vi "13_DC Motor_cts2cm.vi"() -> ()   [LabVIEW 2018]
uses:
  <userlib>/KNR OS 4.0 LabVIEW Toolkit/Type Definition/Resource.ctl
  <userlib>/KNR OS 4.0 LabVIEW Toolkit/Type Definition/DC Motor Port.ctl
panel:
  in  "Speed (+-100%)":dbl(slide) scale=-100.0..100.0
  in  "IP":string(combo)="172.22.11.2"
  in  "Port":T1=4 items=["DS1"=4, "DS2"=5, "DS3"=6, "DS4"=7]
  in  "Resource":T2=enum."KNRm_DDDD"
  in  "stop":bool
  in  "Enable Motor":bool
  out "Position cm":dbl
  out "Velocity (cts/sec)":dbl
  in  "Reverse?":bool
  in  "Reset":bool
  # "KNR/KNRm\nPort5=DS1\nPort6=DS2\nPort7=DS3\nPort8=DS4"
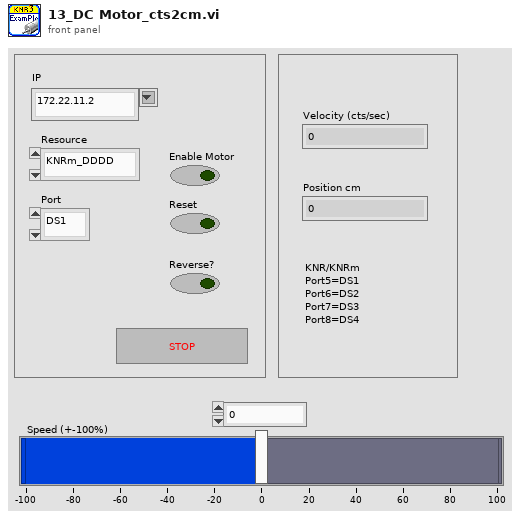
[diagram p1: front panel]
types:
  T1 = typedef "DC Motor Port.ctl" = u16
  T2 = typedef "Resource.ctl" = enum16{"KNRm_DDRC", "KNRm_DDDD", "KNRm_DDDR", "KNRm_DDDC", "KNR", "KNRm_neww"}
  T3 = typedef "KNR3 Reference.ctl" = cluster{"FPGA Session":refnum<class "FPGA Interface Base.lvclass">, "Resource":T2}
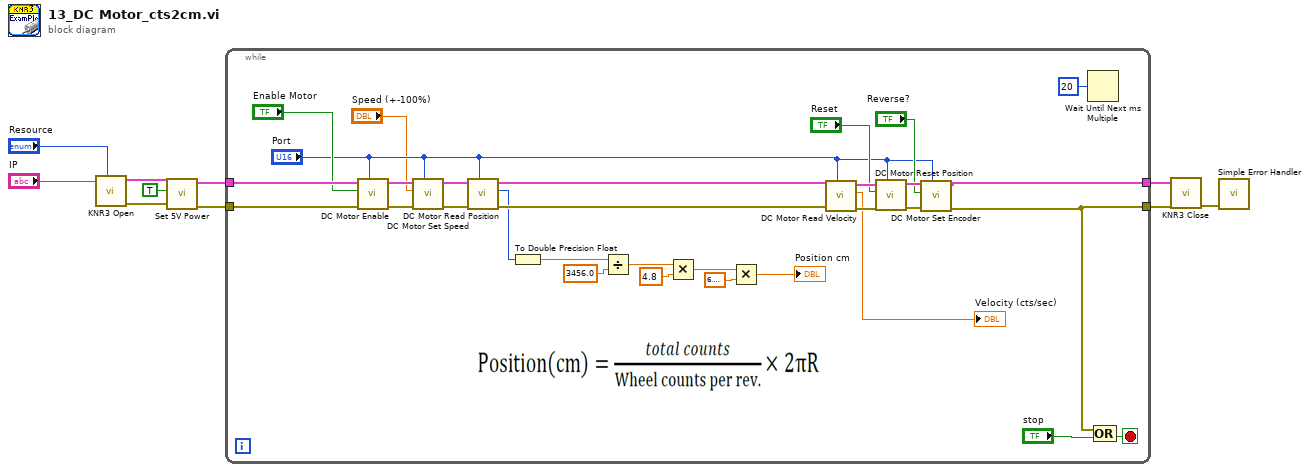
[diagram p0: block diagram]
diagram:
  n1 = call <userlib>:"KNR3 Open.vi"("Resource"="Resource", "IP"="IP") -> ("error out"=w2:errorcluster, "KNR out"=w4:T3)  [unwired: 8 in]
  n2 = call <userlib>:"Set 5V Power.vi"("error in (no error)"=w2, "5V Power(T)"=TRUE ("5V Power"), "KNR in"=w4) -> ("error out"=w8:errorcluster, "KNR out"=w9:T3)  [unwired: 7 in]
  n3 = while {
    tunnel: w9 -> [w41]
    tunnel: w8 -> [w37]
    tunnel: [w26] -> w6
    tunnel: [w27] -> w7
    stop <- w33 stop-if-true
    n4 = call <userlib>:"DC Motor Enable.vi"("Port (DS1)"="Port", "error in (no error)"=w37, "Enable Motor(F)"="Enable Motor", "KNR in"=w41) -> ("error out"=w36:errorcluster, "KNR out"=w40:T3)  [unwired: 6 in]
    n5 = call <userlib>:"DC Motor Set Speed.vi"("Port (DS1)"="Port", "error in (no error)"=w36, "Speed (+-100%)"="Speed (+-100%)", "KNR in"=w40) -> ("error out"=w35:errorcluster, "KNR out"=w39:T3)  [unwired: 6 in]
    n6 = call <userlib>:"DC Motor Read Position.vi"("Port (DS1)"="Port", "error in (no error)"=w35, "KNR in"=w39) -> ("error out"=w30:errorcluster, "Position"=w13:i32, "KNR out"=w31:T3)  [unwired: 6 in]
    n7 = To Double Precision Float(number=w13) -> (double precision float=w12:dbl)
    n8 = Divide(x=w12, y=3456.0) -> (x/y=w17:dbl)
    n9 = Multiply(x=w17, y=4.8 ("x")) -> (x*y=w16:dbl)
    n10 = Multiply(x=w16, y=6.283185307179586) -> (x*y=→"Position cm":dbl)
    n11 = call <userlib>:"DC Motor Read Velocity.vi"("Port (DS1)"="Port", "error in (no error)"=w30, "KNR in"=w31) -> ("error out"=w24:errorcluster, "Velocity (cts/sec)"=→"Velocity (cts/sec)":dbl, "KNR out"=w29:T3)  [unwired: 6 in]
    n12 = call <userlib>:"DC Motor Reset Position.vi"("Port (DS1)"="Port", "error in (no error)"=w24, "Reset(F)"="Reset", "KNR in"=w29) -> ("error out"=w25:errorcluster, "KNR out"=w28:T3)  [unwired: 6 in]
    n13 = call <userlib>:"DC Motor Set Encoder.vi"("Port (DS1)"="Port", "error in (no error)"=w25, "Reverse?(F)"="Reverse?", "KNR in"=w28) -> ("error out"=w26:errorcluster, "KNR out"=w27:T3)  [unwired: 6 in]
    n14 = Wait Until Next ms Multiple(millisecond multiple=u32 20) -> ()  [unwired: 1 out]
    n15 = Compound Arithmetic op=OR(w26, "stop") -> (w33:bool)
  }
  n16 = call <userlib>:"KNR3 Close.vi"("error in (no error)"=w6, "KNR in"=w7) -> ("error out"=w5:errorcluster)  [unwired: 9 in]
  n17 = call <vilib>:"Simple Error Handler.vi"("error in (no error)"=w5) -> ()  [unwired: 4 in, 5 out]
